vi "Intake.vi"(1 "Buttons":bool[](array[boolean])) -> ()   [LabVIEW 2015]
uses:
  Utilities/MotorPositionGlobals.vi
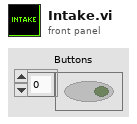
[diagram p1: front panel]
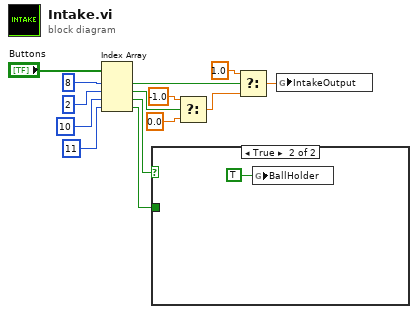
[diagram p0: block diagram]
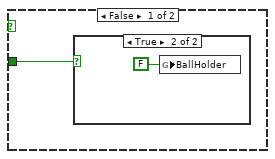
[diagram p2: hidden frame]
diagram:
  n1 = Index Array(array="Buttons", index #1=8 ("index"), index #2=2 ("index"), index #3=10 ("index"), index #4=11 ("index")) -> (element #1=w7:bool, element #2=w6:bool, element #3=w2:bool, element #4=w1:bool)
  n2 = case shown="True" w2 {
    tunnel: w1 -> [w15 _]
    frame False {
      n3 = case shown="True" w15 {
        frame False {
        }
        frame True {
          n4 = global write "MotorPositionGlobals.vi" "BallHolder"(FALSE ("BallHolder")) -> ()
        }
      }
    }
    frame True {
      n5 = global write "MotorPositionGlobals.vi" "BallHolder"(TRUE ("BallHolder")) -> ()
    }
  }
  n6 = Select(t=-1.0, s=w6, f=0.0) -> (s? t:f=w10:dbl)
  n7 = Select(t=1.0, s=w7, f=w10) -> (s? t:f=w5:dbl)
  n8 = global write "MotorPositionGlobals.vi" "IntakeOutput"(w5) -> ()
